vi "Errors.vi"() -> (0 "Errors":T1={"Invalid average number of points"={"status"=TRUE, "code"=5300, "source"="Average number of points cannot be zero"}, "Invalid rate"={"status"=TRUE, "code"=5301, "source"="Rate cannot be zero."}}, 1 "code array":i32[](array[numeric])=[5300, 5301], 2 "description array":string[](array[string])=["Average number of points cannot be zero", "Rate cannot be zero."], 3 "status array":bool[](array[boolean])=[TRUE, TRUE])   [LabVIEW 2017]
uses:
  Controls/Errors.ctl
panel:
  in  "Enum":enum16{"Invalid average number of points"}(ring)
  out "name array":string[](array[string])=["Average number of points cannot be zero", "Rate cannot be zero."]
  in  "Define custom errors here":T1={"Invalid average number of points"={"status"=TRUE, "code"=5300, "source"="Average number of points cannot be zero.\n(Set parameters.vi)"}, "Invalid rate"={"status"=TRUE, "code"=5301, "source"="Rate cannot be zero.\n(Set parameters.vi)"}}
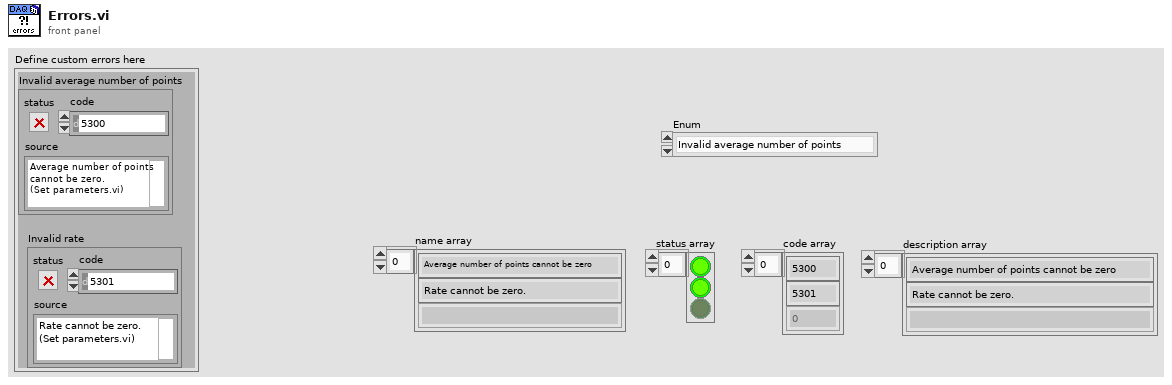
[diagram p1: front panel]
types:
  T1 = typedef "Errors.ctl" = cluster{"Invalid average number of points":errorcluster, "Invalid rate":errorcluster}
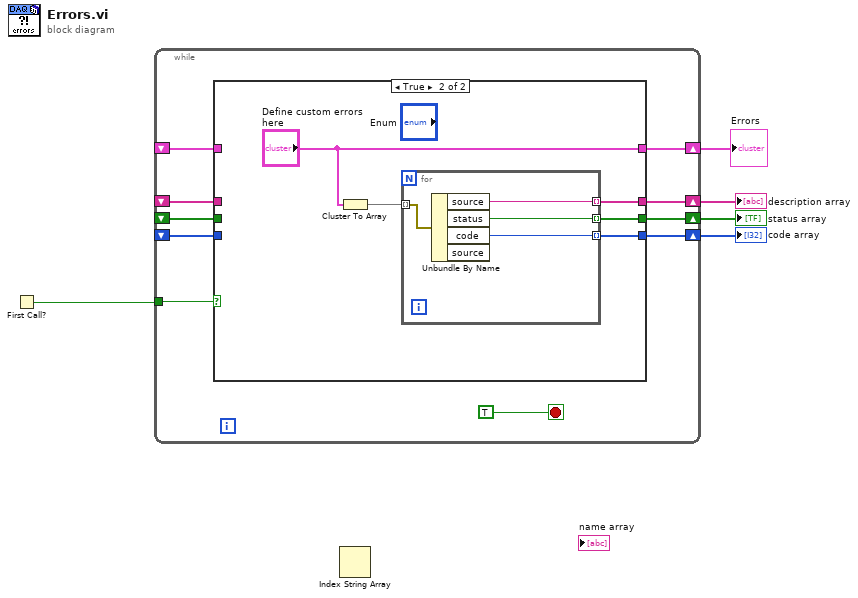
[diagram p0: block diagram]
diagram:
  n1 = First Call?() -> (First Call?: T/F=w5:bool)
  n2 = while {
    shift-right: [w15] -> w2
    shift-left: _ -> [w10]
    shift-right: [w14] -> w1
    shift-left: _ -> [w9]
    shift-right: [w13] -> w3
    shift-left: _ -> [w8]
    tunnel: w5 -> [w11]
    shift-right: [w7] -> w4
    shift-left: _ -> [w6]
    stop <- TRUE stop-if-true
    n3 = case shown="True" w11 {
      tunnel: [w19 w24] -> w15
      tunnel: [w18 w23] -> w14
      tunnel: [w17 w20] -> w13
      tunnel: w10 -> [w19 _]
      tunnel: w9 -> [w18 _]
      tunnel: w8 -> [w17 _]
      tunnel: [w16 "Define custom errors here"] -> w7
      tunnel: w6 -> [w16 _]
      frame False {
      }
      frame True {
        n4 = Cluster To Array(cluster="Define custom errors here") -> (array=w22:errorcluster[])
        n5 = for {
          tunnel: w22 -> [w26] mode=indexing
          tunnel: [w28] -> w23 mode=indexing
          tunnel: [w27] -> w24 mode=indexing
          tunnel: [w25] -> w20 mode=indexing
          n6 = Unbundle By Name(w26) -> ("source"=w25:string, "status"=w27:bool, "code"=w28:i32)  [unwired: 1 out]
        }
      }
    }
  }
  "status array" <- w2
  "code array" <- w1
  "description array" <- w3
  "Errors" <- w4
  n7 = Index String Array() -> ()  [unwired: 3 in, 1 out]
